vi "Calc_Distance_Angle.vi"(0 "X Centroid":dbl=109.0516647531573, 1 "Y Centroid":dbl=88.79391504018369, 2 "X Res":i32=240, 3 "Y Res":i32=320, 4 "Half Horizontal View Angle":dbl=20.25, 5 "Half Vertical View Angle":dbl=27.0, 6 "Camera Height":dbl=44.5, 7 "Target Height":dbl=109.0, 10 "Horizontal Angle Offset":dbl, 11 "Vertical Angle Offset":dbl=4.39) -> (17 "Horizontal Pixel Offset":dbl=-10.948335246842703, 21 "Horizontal Angle":dbl=-1.8475315729047062, 24 "Vertical Angle":dbl=12.016026836969003, 26 "Target Dist":dbl=303.0318149648792)   [LabVIEW 2011]
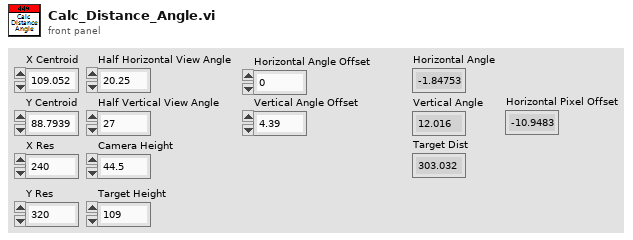
[diagram p1: front panel]
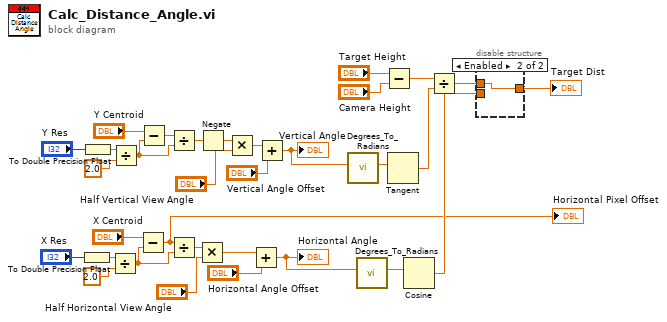
[diagram p0: block diagram]
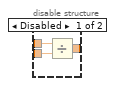
[diagram p2: hidden frame]
diagram:
  n1 = To Double Precision Float(number="X Res") -> (double precision float=w30:dbl)
  n2 = To Double Precision Float(number="Y Res") -> (double precision float=w26:dbl)
  n3 = Divide(x=w30, y=2.0) -> (x/y=w5:dbl)
  n4 = Divide(x=w26, y=2.0) -> (x/y=w7:dbl)
  n5 = Subtract(x="X Centroid", y=w5) -> (x-y=w2:dbl)
  "Horizontal Pixel Offset" <- w2
  n6 = Subtract(x="Y Centroid", y=w7) -> (x-y=w8:dbl)
  n7 = Divide(x=w8, y=w7) -> (x/y=w9:dbl)
  n8 = Divide(x=w2, y=w5) -> (x/y=w6:dbl)
  n9 = Multiply(x=w6, y="Half Horizontal View Angle") -> (x*y=w23:dbl)
  n10 = Negate(x=w9) -> (-x=w21:dbl)
  n11 = Multiply(x=w21, y="Half Vertical View Angle") -> (x*y=w19:dbl)
  n12 = Add(x=w23, y="Horizontal Angle Offset") -> (x+y=w11:dbl)
  "Horizontal Angle" <- w11
  n13 = Add(x=w19, y="Vertical Angle Offset") -> (x+y=w14:dbl)
  "Vertical Angle" <- w14
  n14 = call "Degrees_To_Radians.vi"("Degrees"=w14) -> ("Radians"=w13:dbl)  [unwired: 10 in]
  n15 = call "Degrees_To_Radians.vi"("Degrees"=w11) -> ("Radians"=w4:dbl)  [unwired: 10 in]
  n16 = Subtract(x="Target Height", y="Camera Height") -> (x-y=w15:dbl)
  n17 = Tangent(1:w13) -> (0:w12:dbl)
  n18 = Cosine(x=w4) -> (cos(x)=w10:dbl)
  n19 = Divide(x=w15, y=w12) -> (x/y=w3:dbl)
  n20 = disable-structure shown="Enabled" {
    disable-tunnel: w10 -> [w35 _]
    disable-tunnel: w3 -> [w34 w36]
    disable-tunnel: [w33 w36] -> w1
    frame Disabled {
      n21 = Divide(x=w34, y=w35) -> (x/y=w33:dbl)
    }
    frame Enabled {
    }
  }
  "Target Dist" <- w1
